vi "Periodic Tasks.vi"(8 "error in":errorcluster) -> ()   [LabVIEW 2015]
doc: "This VI runs in parallel to other tasks. It can contain as many user-defined periodic loops as you need. These can carry out PID or other sorts of timed response."
uses:
  Robot Global Data.vi
  <vilib>/addons/control/pid/pid.llb/PID (DBL).vi
  <vilib>/addons/control/pid/NI_PID_pid.lvlib
panel:
  in  "Left D":dbl=20.0
  in  "Left I":dbl=5e-07
  in  "Left P":dbl=0.4
  in  "Right D":dbl=20.0
  in  "Right I":dbl=5e-07
  in  "Right P":dbl=0.4
  in  "Gyro PID Gains":T1={"proportional gain (Kc)"=1.0, "integral time (Ti, min)"=0.0, "derivative time (Td, min)"=0.0} {"derivative time (Td, min)" format="%.3f"; "integral time (Ti, min)" format="%.3f"; "proportional gain (Kc)" format="%.3f"}
  in  "Gyro PID Output":cluster{"output high":dbl, "output low":dbl}={"output high"=100.0, "output low"=-100.0} {"output low" format="%.2f"; "output high" format="%.2f"}
  out "Request Vision Packet":bool
  out "Bytes Written":u32
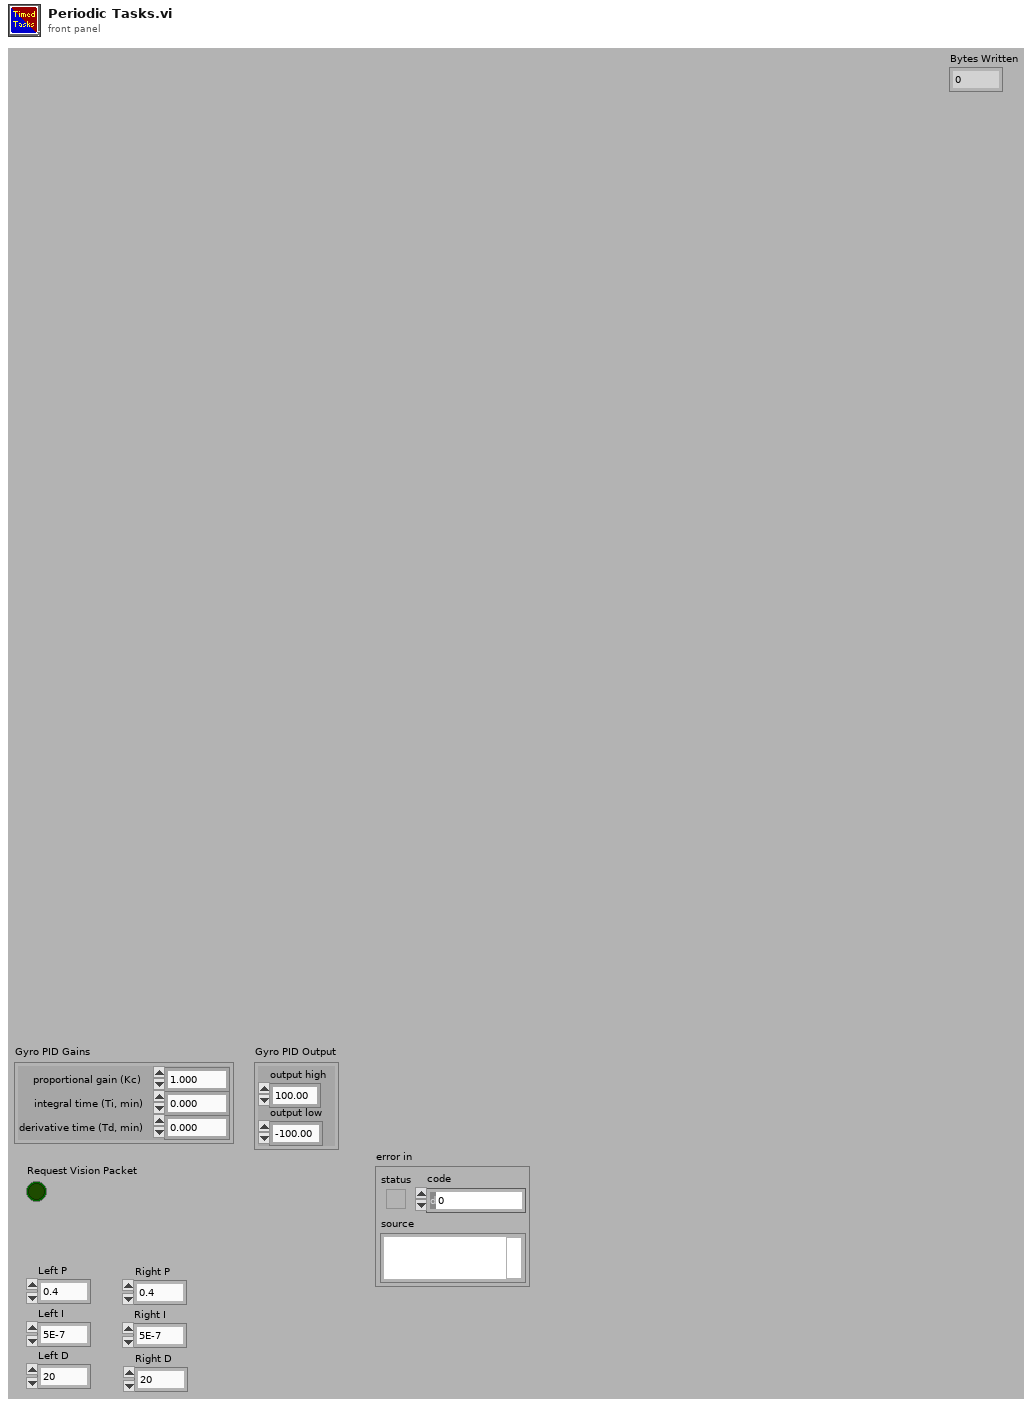
[diagram p1: front panel]
types:
  T1 = cluster{"proportional gain (Kc)":dbl, "integral time (Ti, min)":dbl, "derivative time (Td, min)":dbl}
  T2 = typedef "WPI_DigitalInputDevRef.ctl" = cluster{"DevStatus":errorcluster, "DIO Channel":T3}
  T3 = typedef "FPGA_DIOChannel.ctl" = enum8{"DIO 0", "DIO 1", "DIO 2", "DIO 3", "DIO 4", "DIO 5", "DIO 6", "DIO 7", "DIO 8", "DIO 9", "DIO MXP 0", "DIO MXP 1", "DIO MXP 2", "DIO MXP 3", "DIO MXP 4", "DIO MXP 5", "DIO MXP 6", "DIO MXP 7", "DIO MXP 8", "DIO MXP 9", "DIO MXP 10", "DIO MXP 11", "DIO MXP 12", "DIO MXP 13", "DIO MXP 14", "DIO MXP 15", "Invalid"}
  T4 = typedef "WPI_MotorControlDeviceRef.ctl" = cluster{"DeviceStatus":errorcluster, "Type":T5, "PWM":cluster{"PWM Channel":T6, "DeadBand":T7}, "CAN":cluster{"Device Number":u8, "Control Mode":T8, "Semaphore":T9, "Max Vout":dbl, "TalonSRX Control Mode":T10}, "Invert":bool}
  T5 = typedef "WPI_MotorControlType.ctl" = enum16{"PWM", "CAN", "CANTalonSRX"}
  T6 = typedef "FPGA_DIOPWMChannel.ctl" = enum8{"PWM 0", "PWM 1", "PWM 2", "PWM 3", "PWM 4", "PWM 5", "PWM 6", "PWM 7", "PWM 8", "PWM 9", "PWM MXP 0", "PWM MXP 1", "PWM MXP 2", "PWM MXP 3", "PWM MXP 4", "PWM MXP 5", "PWM MXP 6", "PWM MXP 7", "PWM MXP 8", "PWM MXP 9", "Invalid"}
  T7 = typedef "WPI_PWMDeadband.ctl" = cluster{"Name":string, "maxPositivePwm":i32, "minPositivePwm":i32, "centerPwm":i32, "maxNegativePwm":i32, "minNegativePwm":i32, "angularRange":u16}
  T8 = typedef "WPI_CANJaguar_ControlMode.ctl" = enum8{"Percent VBus", "Current", "Speed", "Position", "Voltage"}
  T9 = typedef "Semaphore RefNum" = refnum<k1>
  T10 = typedef "WPI_CANTalonSRX_APIControlMode.ctl" = enum8{"Percent VBus", "Speed", "Position", "Slave", "Unchanged / Invalid", "Voltage Compensation", "Current", "Motion Profile"}
  T11 = typedef "WPI_SerialPortRef.ctl" = cluster{"DevStatus":errorcluster, "Serial Port Name":refnum<visa-resource-name>}
  T12 = typedef "WPI_GyroDevRef.ctl" = cluster{"DevStatus":errorcluster, "Analog Channel":T13, "Offset":dbl, "Gain (VoltsPerDegree/Second)":dbl, "Gyro Type":enum16{"Analog", "XRS450"}, "Handle":i32, "SPI Bus":T14, "Device Found":bool, "Sample Rate":dbl, "Calibrate On Open":bool}
  T13 = typedef "FPGA_AIChannel.ctl" = enum8{"AI 0", "AI 1", "AI 2", "AI 3", "AI MXP 0", "AI MXP 1", "AI MXP 2", "AI MXP 3", "Invalid"}
  T14 = typedef "spi_bus.ctl" = enum16{"SPI On-Board, CS0", "SPI On-Board, CS1", "SPI On-Board, CS2", "SPI On-Board, CS3", "SPI MXP", "Invalid"}
  T15 = cluster{"y":dbl, "distance":dbl, "angle":dbl, "goal":bool, "x":dbl}
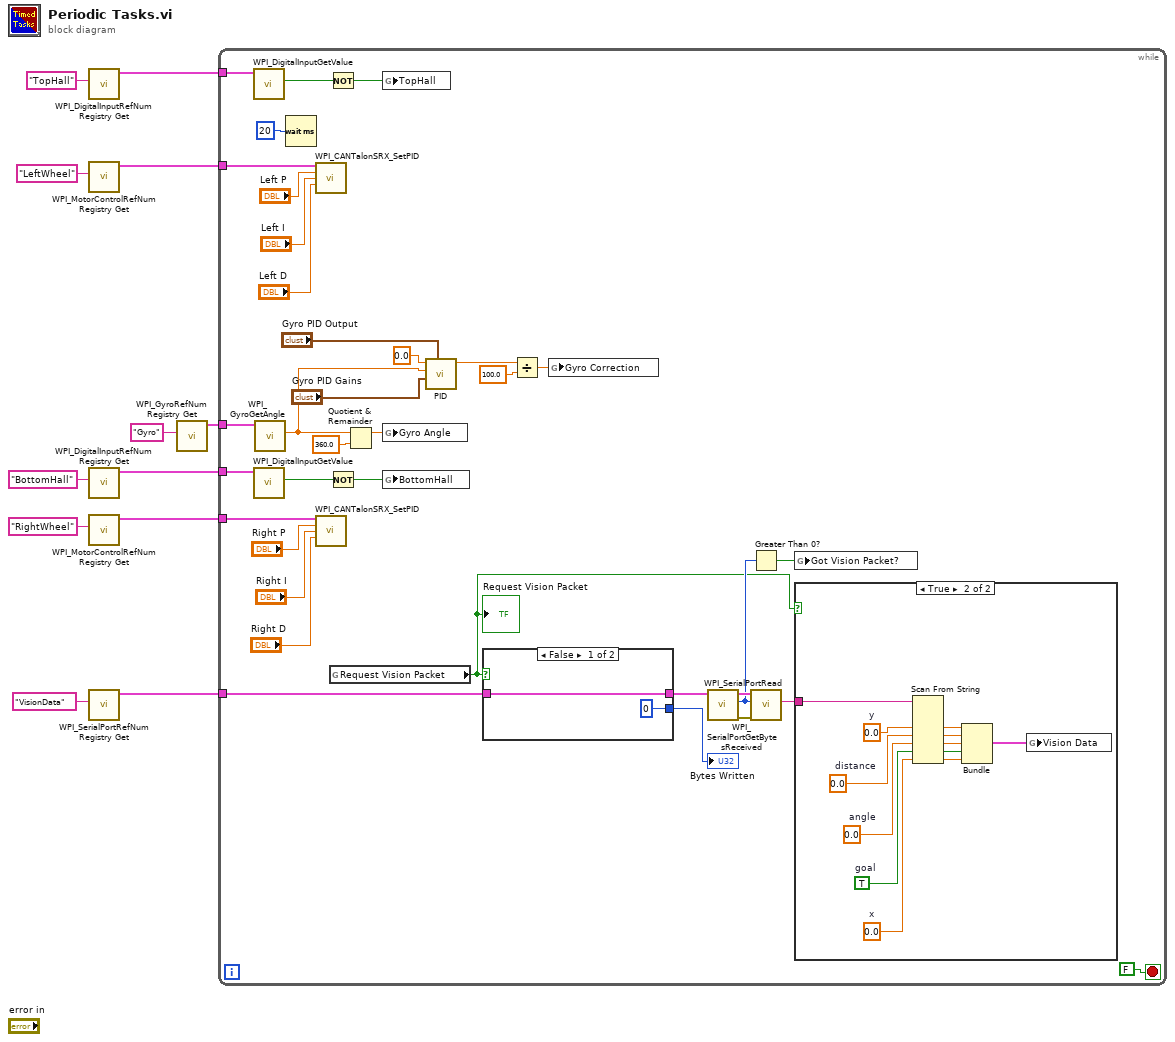
[diagram p0: block diagram]
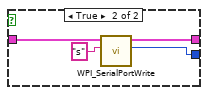
[diagram p3: hidden frame]
diagram:
  n1 = call <vilib>:"WPI_DigitalInputRefNum Registry Get.vi"("refnum name"="TopHall") -> ("DigitalInputDevRef"=w6:T2)  [unwired: 9 in, 1 out]
  n2 = call <vilib>:"WPI_MotorControlRefNum Registry Get.vi"("refnum name"="LeftWheel") -> ("MotorControlDevRef"=w3:T4)  [unwired: 9 in, 1 out]
  n3 = call <vilib>:"WPI_DigitalInputRefNum Registry Get.vi"("refnum name"="BottomHall") -> ("DigitalInputDevRef"=w4:T2)  [unwired: 9 in, 1 out]
  n4 = call <vilib>:"WPI_MotorControlRefNum Registry Get.vi"("refnum name"="RightWheel") -> ("MotorControlDevRef"=w5:T4)  [unwired: 9 in, 1 out]
  n5 = call <vilib>:"WPI_SerialPortRefNum Registry Get.vi"("refnum name"="VisionData") -> ("SerialPortRef"=w1:T11)  [unwired: 9 in, 1 out]
  n6 = call <vilib>:"WPI_GyroRefNum Registry Get.vi"("refnum name"="Gyro") -> ("GyroDevRef"=w2:T12)  [unwired: 9 in, 1 out]
  n7 = while {
    tunnel: w6 -> [w18]
    tunnel: w5 -> [w17]
    tunnel: w4 -> [w16]
    tunnel: w3 -> [w15]
    tunnel: w2 -> [w14]
    tunnel: w1 -> [w13]
    stop <- FALSE stop-if-true
    n8 = call <vilib>:"WPI_DigitalInputGetValue.vi"("DigitalInputDevRef"=w18) -> ("Value"=w21:bool)  [unwired: 8 in, 2 out]
    n9 = call <vilib>:"WPI_DigitalInputGetValue.vi"("DigitalInputDevRef"=w16) -> ("Value"=w22:bool)  [unwired: 8 in, 2 out]
    n10 = call <vilib>:"WPI_GyroGetAngle.vi"("GyroDevRef"=w14) -> ("Angle"=w35:dbl)  [unwired: 6 in, 4 out]
    n11 = Wait (ms)(milliseconds to wait=u32 20) -> ()  [unwired: 1 out]
    n12 = call <vilib>:"WPI_CANTalonSRX_SetPID.vi"("CAN Talon SRX Ref"=w15, "P"="Left P", "I"="Left I", "D"="Left D") -> ()  [unwired: 10 in, 2 out]
    n13 = call <vilib>:"WPI_CANTalonSRX_SetPID.vi"("CAN Talon SRX Ref"=w17, "P"="Right P", "I"="Right I", "D"="Right D") -> ()  [unwired: 10 in, 2 out]
    n14 = Not(x=w21) -> (.not. x?=w20:bool)
    n15 = Not(x=w22) -> (.not. x?=w19:bool)
    n16 = global read "Robot Global Data.vi" "Request Vision Packet"() -> (w39:bool)
    "Request Vision Packet" <- w39
    n17 = Quotient & Remainder(x=w35, y=360.0) -> (x-y*floor(x/y)=w36:dbl)  [unwired: 1 out]
    n18 = global write "Robot Global Data.vi" "TopHall"(w20) -> ()
    n19 = global write "Robot Global Data.vi" "Gyro Angle"(w36) -> ()
    n20 = global write "Robot Global Data.vi" "BottomHall"(w19) -> ()
    n21 = call-poly <vilib>:"PID.vi"("output range"="Gyro PID Output", "PID gains"="Gyro PID Gains", "process variable"=w35, "setpoint"=0.0) -> ("output"=w31:dbl)  [unwired: 6 in, 1 out]
    n22 = case shown="False" w39 {
      tunnel: [w60 w64] -> w43
      tunnel: [u32 0 ("Num Bytes Written") w63] -> w42
      tunnel: w13 -> [w60 w62]
      frame False {
      }
      frame True {
        n23 = call <vilib>:"WPI_SerialPortWrite.vi"("Buffer"="s", "SerialPortRef"=w62) -> ("Num Bytes Written"=w63:u32, "SerialPortRef"=w64:T11)  [unwired: 7 in, 1 out]
      }
    }
    "Bytes Written" <- w42
    n24 = Divide(x=w31, y=100.0) -> (x/y=w32:dbl)
    n25 = global write "Robot Global Data.vi" "Gyro Correction"(w32) -> ()
    n26 = call <vilib>:"WPI_SerialPortGetBytesReceived.vi"("SerialPortRef"=w43) -> ("error out"=w44:errorcluster, "Bytes at Port"=w41:u32, "SerialPortRef"=w45:T11)  [unwired: 8 in]
    n27 = Greater Than 0?(x=w41) -> (x > 0?=w40:bool)
    n28 = call <vilib>:"WPI_SerialPortRead.vi"("error in (no error)"=w44, "Num Bytes to Read"=w41, "SerialPortRef"=w45) -> ("Buffer"=w38:string)  [unwired: 6 in, 2 out]
    n29 = global write "Robot Global Data.vi" "Got Vision Packet?"(w40) -> ()
    n30 = case shown="True" w39 {
      tunnel: w38 -> [_ w48]
      frame False {
      }
      frame True {
        w56 = TRUE  # goal
        w55 = 0.0  # x
        w57 = 0.0  # angle
        w58 = 0.0  # distance
        w59 = 0.0  # y
        n31 = Scan From String(input string=w48, default 1=w59, default 2=w58, default 3=w57, default 4=w56, default 5=w55) -> (output 1=w54:dbl, output 2=w53:dbl, output 3=w52:dbl, output 4=w51:bool, output 5=w50:dbl)  [unwired: 3 in, 3 out]
        n32 = Bundle("y"=w54, "distance"=w53, "angle"=w52, "goal"=w51, "x"=w50) -> (w49:T15)  [unwired: 1 in]
        n33 = global write "Robot Global Data.vi" "Vision Data"(w49) -> ()
      }
    }
  }
